vi "Read Sensor metadata.vi"(11 "Template in":refnum<class "Template.lvclass">) -> (3 "Sensor Data":u8[](array[numeric]))   [LabVIEW 2020, in "Template.lvlib" / "Template.lvclass"]
uses:
  Template.lvclass
  Template.lvclass/Template.ctl
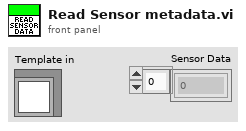
[diagram p1: front panel]
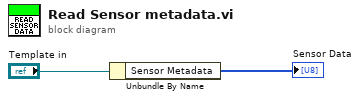
[diagram p0: block diagram]
diagram:
  n1 = Unbundle By Name("Template in") -> ("Sensor Metadata"=→"Sensor Data":u8[])
